vi "table using for loop.vi"() -> ()   [LabVIEW 2020]
panel:
  out "Array 2":dbl[][](array[numeric])
  out "Array":dbl[](array[numeric])
  in  "Numeric":dbl
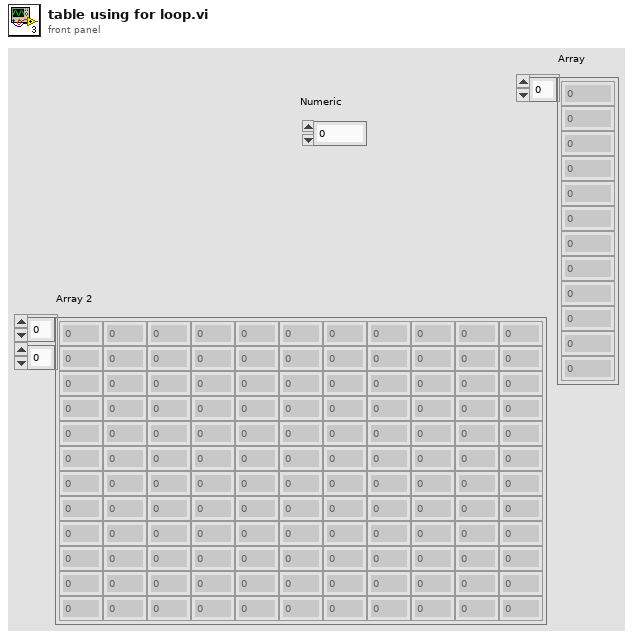
[diagram p1: front panel]
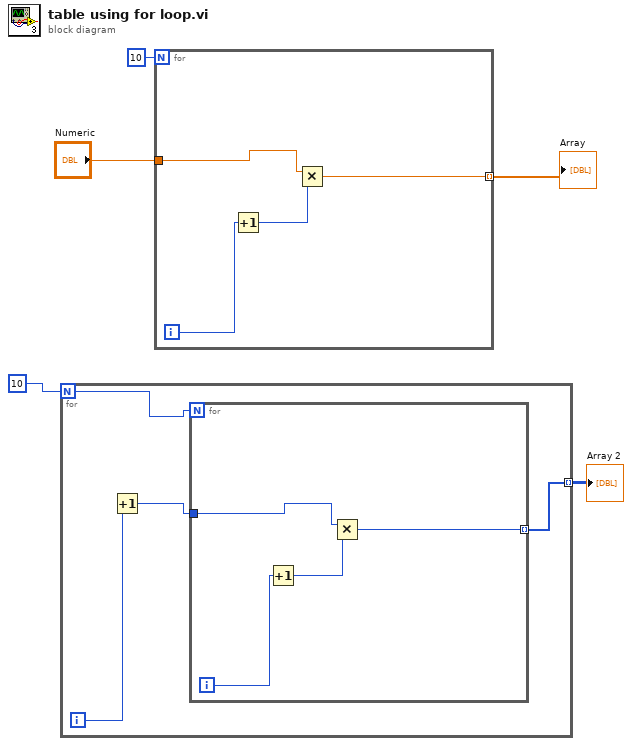
[diagram p0: block diagram]
diagram:
  n1 = for {
    N: 10 -> [w7]
    tunnel: [w6] -> w1 mode=indexing
    i -> [w9]
    n2 = Increment(x=w9) -> (x+1=w8:i32)
    n3 = for {
      N: w7 -> [_]
      tunnel: w8 -> [w13]
      tunnel: [w10] -> w6 mode=indexing
      i -> [w12]
      n4 = Increment(x=w12) -> (x+1=w11:i32)
      n5 = Multiply(x=w13, y=w11) -> (x*y=w10:i32)
    }
  }
  "Array 2" <- w1
  n6 = for {
    N: 10 -> [_]
    tunnel: "Numeric" -> [w17]
    tunnel: [w14] -> w3 mode=indexing
    i -> [w16]
    n7 = Increment(x=w16) -> (x+1=w15:i32)
    n8 = Multiply(x=w17, y=w15) -> (x*y=w14:dbl)
  }
  "Array" <- w3
